vi "Translator SD Card Library.vi"(0 "Input":variant=variant("Function Name"=variant(string "Strip Path"), "Input Datatypes"=variant(string[] ["error", "int"]), "Inputs"=variant(string[] ["error in", "x"]), "Node refnum"=variant(refnum<vi> refnum), "Output Datatypes"=variant(string[] ["int"]), "Outputs"=variant(string[] ["a"])), 11 "error in (no error)":errorcluster) -> (4 "Output":variant=variant("Defines"=variant(string[] []), "Includes"=variant(string[] []), "Replaced Code"=variant(string "/* LabVIEW system function 'Strip Path' not found. */")), 15 "error out":errorcluster)   [LabVIEW 2014, in "LabVIEW Universal Transcriptor SD Card Library.lvlib"]
doc: "Translator for SD card. This library is inteded just for one SD card, not multiple, because arduino functios are written over global object, there is no need to have class implementation."
uses:
  LabVIEW Universal Transcriptor SD Card Library.lvlib
panel:
  out "Outputs":string[](array[string])
  out "Inputs":string[](array[string])
  out "Output Datatypes":string[](array[string])
  out "Input Datatypes":string[](array[string])
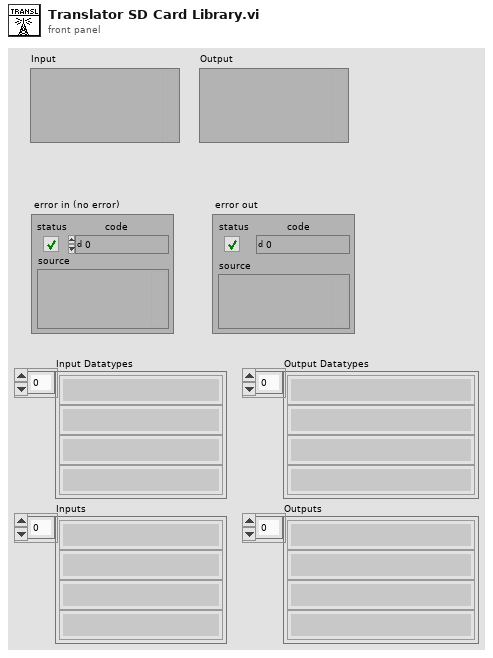
[diagram p1: front panel]
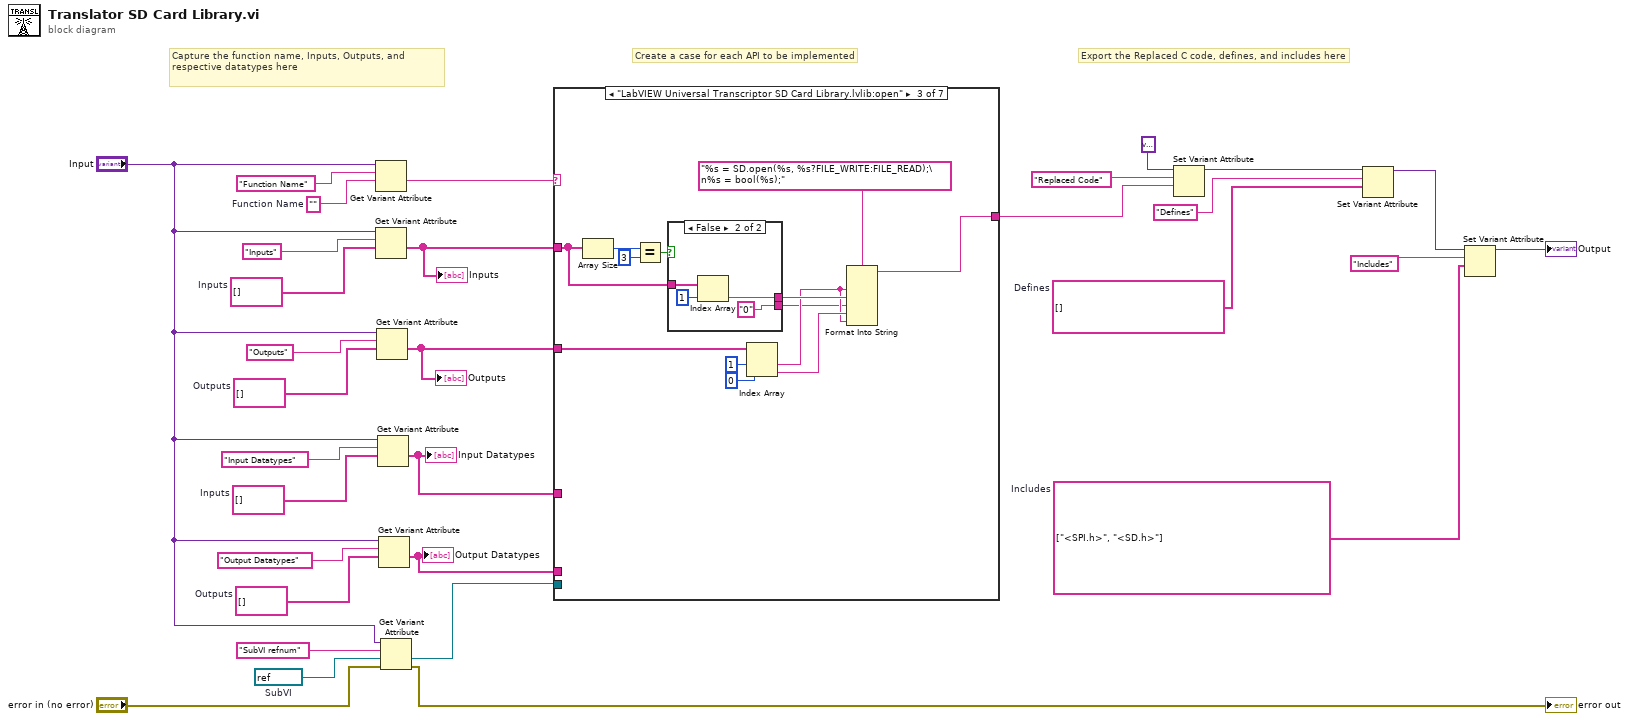
[diagram p0: block diagram]
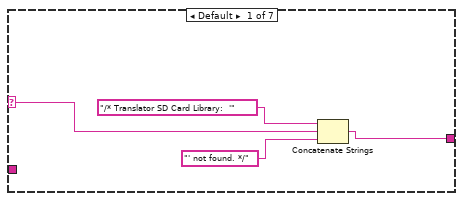
[diagram p2: hidden frame]
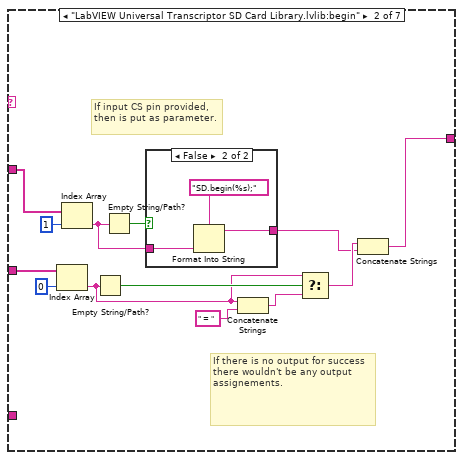
[diagram p3: hidden frame]
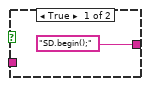
[diagram p4: hidden frame]
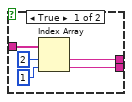
[diagram p5: hidden frame]
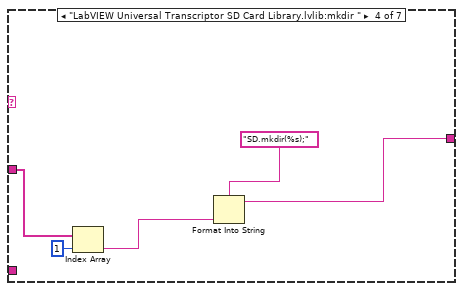
[diagram p6: hidden frame]
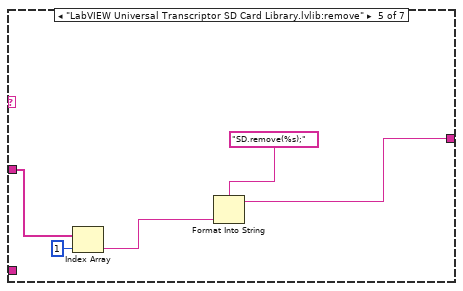
[diagram p7: hidden frame]
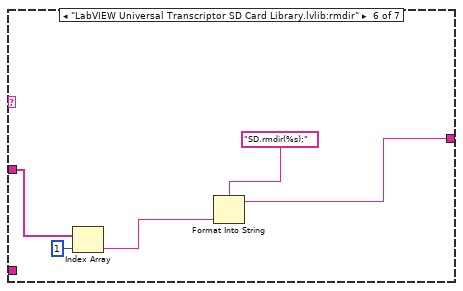
[diagram p8: hidden frame]
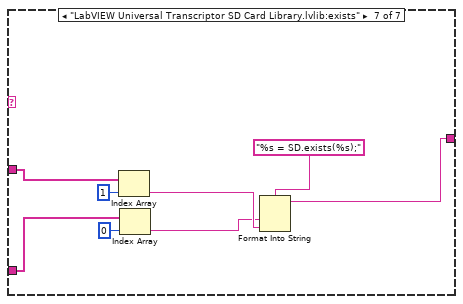
[diagram p9: hidden frame]
diagram:
  w7 = refnum<vi> refnum  # SubVI
  w4 = string[] []  # Defines
  w17 = string[] []  # Outputs
  w18 = string[] []  # Inputs
  w3 = string[] ["<SPI.h>", "<SD.h>"]  # Includes
  w27 = string[] []  # Outputs
  w28 = string[] []  # Inputs
  w29 = ""  # Function Name
  # "Capture the function name, Inputs, Outputs, and respective datatypes here"
  # "Export the Replaced C code, defines, and includes here"
  # "Create a case for each API to be implemented"
  n1 = Get Variant Attribute(Variant="Input", name="Function Name", default value (empty Variant)=w29) -> (value=w24:string)  [unwired: 1 in, 3 out]
  n2 = Get Variant Attribute(Variant="Input", name="Inputs", default value (empty Variant)=w28) -> (value=w14:string[])  [unwired: 1 in, 3 out]
  "Inputs" <- w14
  n3 = Get Variant Attribute(Variant="Input", name="Outputs", default value (empty Variant)=w27) -> (value=w15:string[])  [unwired: 1 in, 3 out]
  "Outputs" <- w15
  n4 = Get Variant Attribute(Variant="Input", name="Input Datatypes", default value (empty Variant)=w18) -> (value=w10:string[])  [unwired: 1 in, 3 out]
  "Input Datatypes" <- w10
  n5 = Get Variant Attribute(Variant="Input", name="Output Datatypes", default value (empty Variant)=w17) -> (value=w5:string[])  [unwired: 1 in, 3 out]
  "Output Datatypes" <- w5
  n6 = Get Variant Attribute(Variant="Input", name="SubVI refnum", default value (empty Variant)=w7, error in="error in (no error)") -> (value=w6:refnum<vi>, error out=→"error out":errorcluster)  [unwired: 2 out]
  n7 = case shown="\"LabVIEW Universal Transcriptor SD Card Library.lvlib:open\"" w24 {
    selector: w24 -> [w34 _ _ _ _ _ _]
    tunnel: [w32 w36 w63 w76 w81 w86 w90] -> w23
    tunnel: w14 -> [_ w43 w57 w75 w80 w85 w94]
    tunnel: w15 -> [_ w45 w64 _ _ _ w92]
    tunnel: w10 -> [_ _ _ _ _ _ _]
    tunnel: w6 -> [_ _ _ _ _ _ _]
    tunnel: w5 -> [_ _ _ _ _ _ _]
    frame Default {
      n8 = Concatenate Strings("/* Translator SD Card Library:  '", w34, "' not found. */") -> (w32:string)
    }
    frame "LabVIEW Universal Transcriptor SD Card Library.lvlib:begin" {
      # "If input CS pin provided, then is put as parameter."
      # "If there is no output for success there wouldn't be any output assignements."
      n9 = Index Array(array=w45, index=0) -> (element=w40:string)
      n10 = Index Array(array=w43, index=1) -> (element=w46:string)
      n11 = Empty String/Path?(string/path=w40) -> (empty?=w42:bool)
      n12 = Empty String/Path?(string/path=w46) -> (empty?=w47:bool)
      n13 = case shown="False" w47 {
        tunnel: w46 -> [_ w51]
        tunnel: ["SD.begin();" w50] -> w37
        frame True {
        }
        frame False {
          n14 = Format Into String(format string="SD.begin(%s);", w51) -> (resulting string=w50:string)  [unwired: 2 in, 1 out]
        }
      }
      n15 = Concatenate Strings(w40, " = " ("string")) -> (w39:string)
      n16 = Select(t=w40, s=w42, f=w39) -> (s? t:f=w38:string)
      n17 = Concatenate Strings(w38, w37) -> (w36:string)
    }
    frame "LabVIEW Universal Transcriptor SD Card Library.lvlib:open" {
      n18 = Array Size(array=w57) -> (size(s)=w56:i32)
      n19 = Equal?(x=w56, y=3) -> (x = y?=w54:bool)
      n20 = case shown="False" w54 {
        tunnel: w57 -> [w69 w73]
        tunnel: [w68 w72] -> w59
        tunnel: [w66 "0" ("element")] -> w53
        frame True {
          n21 = Index Array(array=w69, index #1=2 ("index"), index #2=1 ("index")) -> (element #1=w68:string, element #2=w66:string)
        }
        frame False {
          n22 = Index Array(array=w73, index=1) -> (element=w72:string)
        }
      }
      n23 = Index Array(array=w64, index #1=1 ("index"), index #2=0 ("index")) -> (element #1=w58:string, element #2=w60:string)
      n24 = Format Into String(format string="%s = SD.open(%s, %s?FILE_WRITE:FILE_READ);\n%s = bool(%s);", w58, w59, w53, w60, w58) -> (resulting string=w63:string)  [unwired: 2 in, 1 out]
    }
    frame "LabVIEW Universal Transcriptor SD Card Library.lvlib:mkdir " {
      n25 = Index Array(array=w75, index=1) -> (element=w77:string)
      n26 = Format Into String(format string="SD.mkdir(%s);", w77) -> (resulting string=w76:string)  [unwired: 2 in, 1 out]
    }
    frame "LabVIEW Universal Transcriptor SD Card Library.lvlib:remove" {
      n27 = Index Array(array=w80, index=1) -> (element=w82:string)
      n28 = Format Into String(format string="SD.remove(%s);", w82) -> (resulting string=w81:string)  [unwired: 2 in, 1 out]
    }
    frame "LabVIEW Universal Transcriptor SD Card Library.lvlib:rmdir" {
      n29 = Index Array(array=w85, index=1) -> (element=w87:string)
      n30 = Format Into String(format string="SD.rmdir(%s);", w87) -> (resulting string=w86:string)  [unwired: 2 in, 1 out]
    }
    frame "LabVIEW Universal Transcriptor SD Card Library.lvlib:exists" {
      n31 = Index Array(array=w94, index=1) -> (element=w93:string)
      n32 = Index Array(array=w92, index=0) -> (element=w91:string)
      n33 = Format Into String(format string="%s = SD.exists(%s);", w91, w93) -> (resulting string=w90:string)  [unwired: 2 in, 1 out]
    }
  }
  n34 = Set Variant Attribute(Variant=variant ("variant"), name="Replaced Code", value=w23) -> (Variant out=w13:variant)  [unwired: 1 in, 2 out]
  n35 = Set Variant Attribute(Variant=w13, name="Defines", value=w4) -> (Variant out=w12:variant)  [unwired: 1 in, 2 out]
  n36 = Set Variant Attribute(Variant=w12, name="Includes", value=w3) -> (Variant out=→"Output":variant)  [unwired: 1 in, 2 out]
